vi "Charger_Find All IPGs.vi"(6 "Stop Refnum":refnum<vi>, 7 "IPG Status Array":T1[](array[typedef]), 8 "error in":errorcluster, 9 "MICS Parameters":T2[](array[typedef])=[{"address"="COM11", "chan"=2, "ID"=0}, {"address"="COM12", "chan"=3, "ID"=0}, {"address"="COM13", "chan"=4, "ID"=0}, {"address"="COM14", "chan"=5, "ID"=0}, {"address"="COM15", "chan"=6, "ID"=0}, {"address"="COM16", "chan"=7, "ID"=0}] {"ID" format="%06x"; "chan" min=1 max=10 step=1}, 10 "Charger Setpoint":dbl=7500.0, 11 "Charger COM Port":refnum<visa-resource-name>="COM9") -> (0 "error out":errorcluster)   [LabVIEW 2020]
uses:
  MICS_Input Control.ctl
  Charger_Status Refnum.ctl
  Drivers/Charger Test Set/Charger_Input Control.ctl
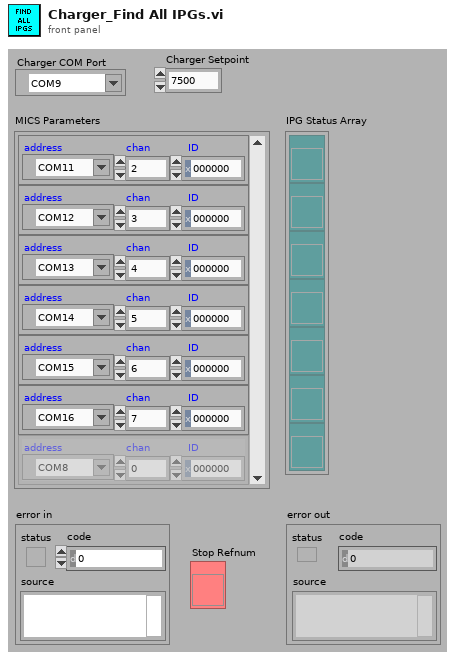
[diagram p1: front panel]
types:
  T1 = typedef "Charger_Status Refnum.ctl" = refnum<vi>
  T2 = typedef "MICS_Input Control.ctl" = cluster{"address":refnum<visa-resource-name>, "chan":u16, "ID":u32}
  T3 = typedef "Charger_Input Control.ctl" = cluster{"address":refnum<visa-resource-name>, "position":i32, "setpoint":dbl}
  T4 = cluster{"MICS ID":u32, "VBAT":dbl, "ChargingState":string, "VBAT Slide":dbl, "Status":string, "TemperatureLevel":dbl, "IPG_ReceivedLevel":dbl, "VBAT Target":dbl, "Charger Setpoint":dbl, "Index":i32, "Ready":bool, "Charger Inputs":T3, "MICS Inputs":cluster{"address":refnum<visa-resource-name>, "chan":u16, "ID":u32}}
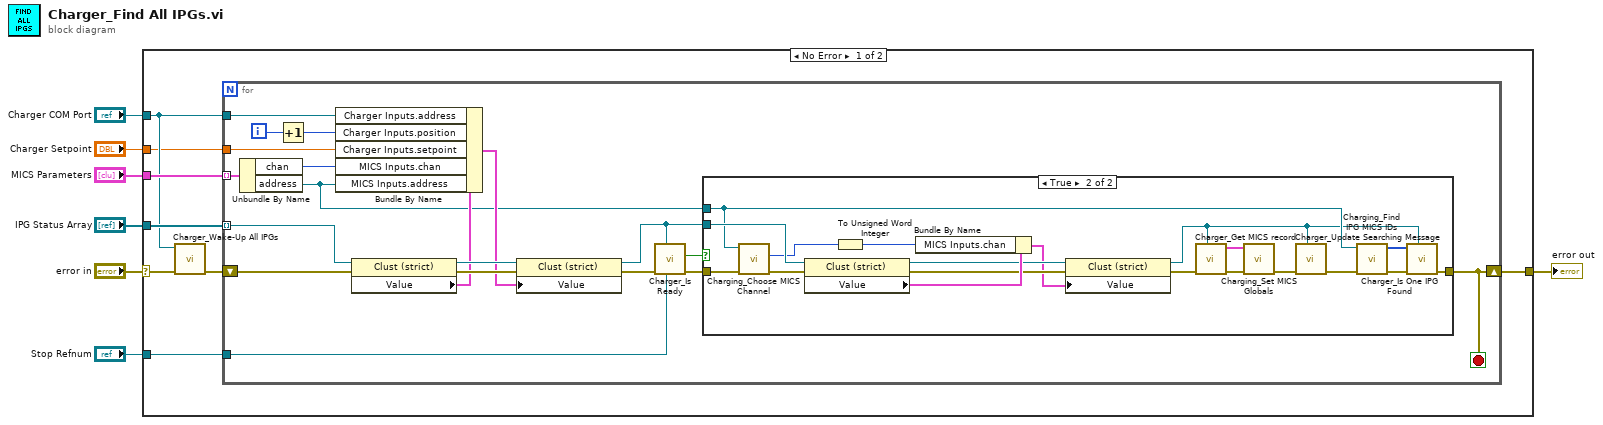
[diagram p0: block diagram]
diagram:
  n1 = case shown="No Error" "error in" {
    selector: "error in" -> [w9 w55]
    tunnel: [w15 w55] -> w7
    tunnel: "MICS Parameters" -> [w13 _]
    tunnel: "IPG Status Array" -> [w12 _]
    tunnel: "Charger COM Port" -> [w11 _]
    tunnel: "Charger Setpoint" -> [w10 _]
    tunnel: "Stop Refnum" -> [w8 _]
    frame No Error {
      n2 = call "Charger_Wake-Up All IPGs.vi"("error in"=w9, "Charger COM Port"=w11) -> ("error out"=w14:errorcluster)  [unwired: 9 in]
      n3 = for {
        shift-right: [w18] -> w15
        shift-left: w14 -> [w31]
        tunnel: w13 -> [w34] mode=indexing
        tunnel: w12 -> [w21] mode=indexing
        tunnel: w11 -> [w29]
        tunnel: w10 -> [w26]
        tunnel: w8 -> [w32]
        i -> [w33]
        stop <- w18 stop-if-true
        n4 = Unbundle By Name(w34) -> ("chan"=w27:u16, "address"=w22:refnum<visa-resource-name>)
        n5 = Increment(x=w33) -> (x+1=w28:i32)
        n6 = property class="Clust (strict)"(reference=w21, error in=w31) -> (reference out=w25:T1, error out=w30:errorcluster, "Value"=w24:T4)
        n7 = Bundle By Name(cluster=w24, "Charger Inputs.address"=w29, "Charger Inputs.position"=w28, "Charger Inputs.setpoint"=w26, "MICS Inputs.chan"=w27, "MICS Inputs.address"=w22) -> (w23:T4)
        n8 = property class="Clust (strict)"(reference=w25, error in=w30, "Value"=w23) -> (reference out=w16:T1, error out=w20:errorcluster)
        n9 = call "Charger_Is Ready.vi"("Stop Refnum"=w32, "Status Refnum"=w16, "error in"=w20) -> ("error out"=w19:errorcluster, "ready"=w17:bool)  [unwired: 7 in]
        n10 = case shown="True" w17 {
          tunnel: w22 -> [_ w41]
          tunnel: w19 -> [w35 w50]
          tunnel: w16 -> [_ w48]
          tunnel: [w35 w52] -> w18
          frame False {
          }
          frame True {
            n11 = call "Charging_Choose MICS Channel.vi"("error in"=w50, "MICS COM port"=w41) -> ("error out"=w49:errorcluster, "Selected MICS Channel"=w46:u8)  [unwired: 6 in]
            n12 = property class="Clust (strict)"(reference=w48, error in=w49) -> (reference out=w43:T1, error out=w44:errorcluster, "Value"=w47:T4)
            n13 = To Unsigned Word Integer(number=w46) -> (unsigned 16bit integer=w45:u16)
            n14 = Bundle By Name(cluster=w47, "MICS Inputs.chan"=w45) -> (w42:T4)
            n15 = property class="Clust (strict)"(reference=w43, error in=w44, "Value"=w42) -> (reference out=w36:T1, error out=w38:errorcluster)
            n16 = call "Charger_Get MICS record.vi"("Status Refnum"=w36, "error in"=w38) -> ("error out"=w39:errorcluster, "MICS Inputs"=w40:T2)  [unwired: 3 in, 3 out]
            n17 = call "Charging_Set MICS Globals.vi"("error in"=w39, "MICS inputs"=w40) -> ("error out"=w37:errorcluster)  [unwired: 4 in, 1 out]
            n18 = call "Charger_Update Searching Message.vi"("Status Refnum"=w36, "error in"=w37) -> ("error out"=w51:errorcluster)  [unwired: 7 in]
            n19 = call "Charging_Find IPG MICS IDs.vi"("error in"=w51, "MICS COM port"=w41) -> ("error out"=w54:errorcluster, "detected MICS IDs"=w53:u32[])  [unwired: 6 in]
            n20 = call "Charger_Is One IPG Found.vi"("Status Refnum"=w36, "error in"=w54, "MICS ID array"=w53) -> ("error out"=w52:errorcluster)  [unwired: 4 in, 2 out]
          }
        }
      }
    }
    frame Error {
    }
  }
  "error out" <- w7
